vi "USRP oneTx_demoinfocom.vi"() -> ()   [LabVIEW 2021]
uses:
  system stop.vi
  <instrlib>/niUSRP/niUSRP Write Tx Data (CDB Cluster).vi
panel:
  out "Waveform Graph":dbl[](graph)
  in  "Duration":dbl format="%#_13g"
  in  "Frequency":dbl format="%#_13g"
  out "coerced carrier frequency":dbl=100000.0 format="%#_6p"
  out "coerced IQ rate":dbl=100000.0 format="%#_6p"
  in  "Tx IP":refnum<k15>
  in  "Tx Gain":dbl format="%#_6f"
  in  "carrier frequency":dbl=100000.0 format="%#_6p"
  in  "IQ rate":dbl=100000.0 format="%#_6p"
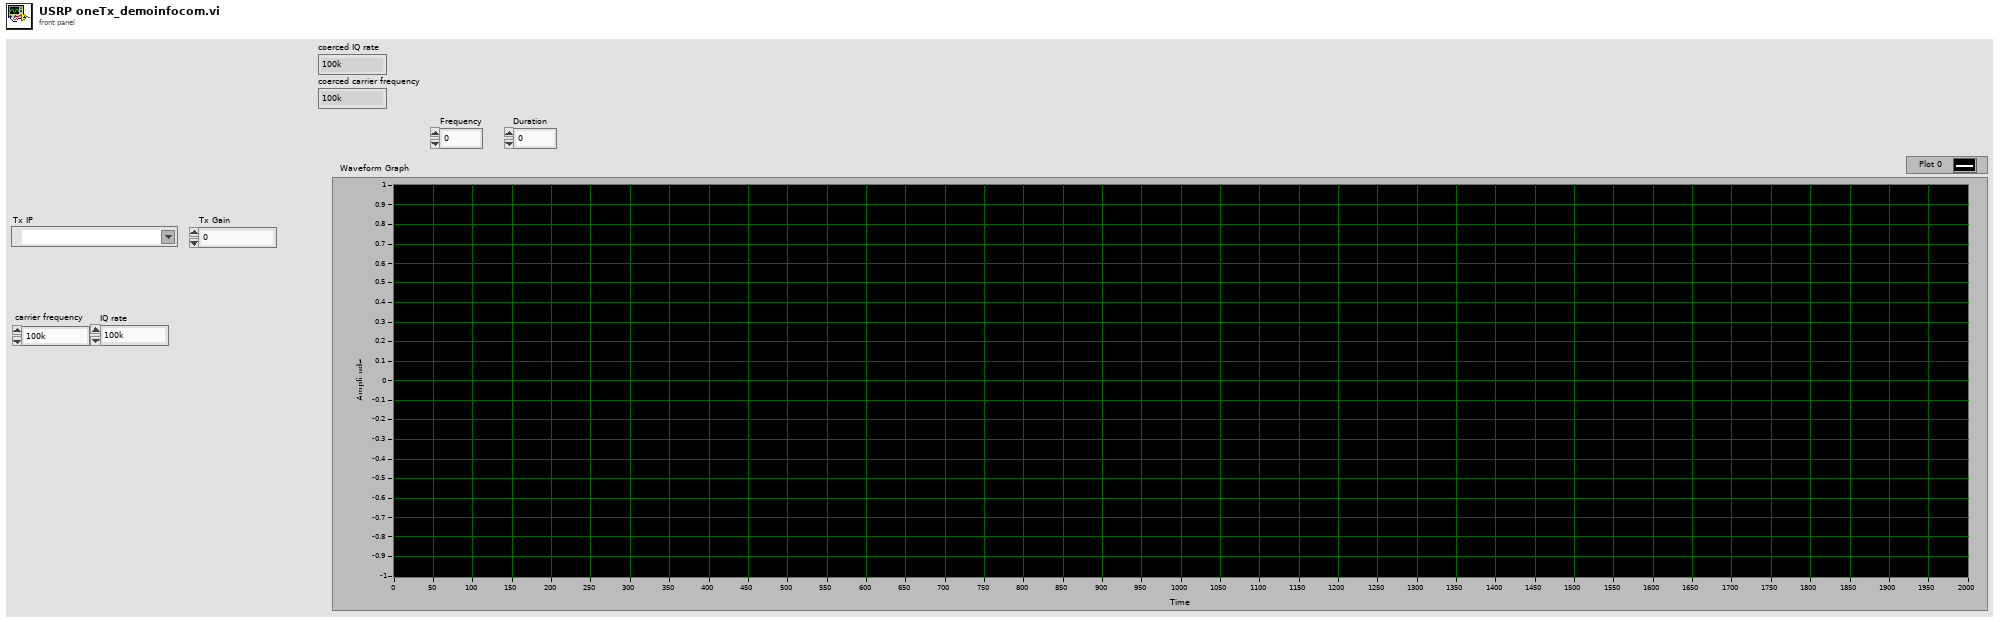
[diagram p1: front panel]
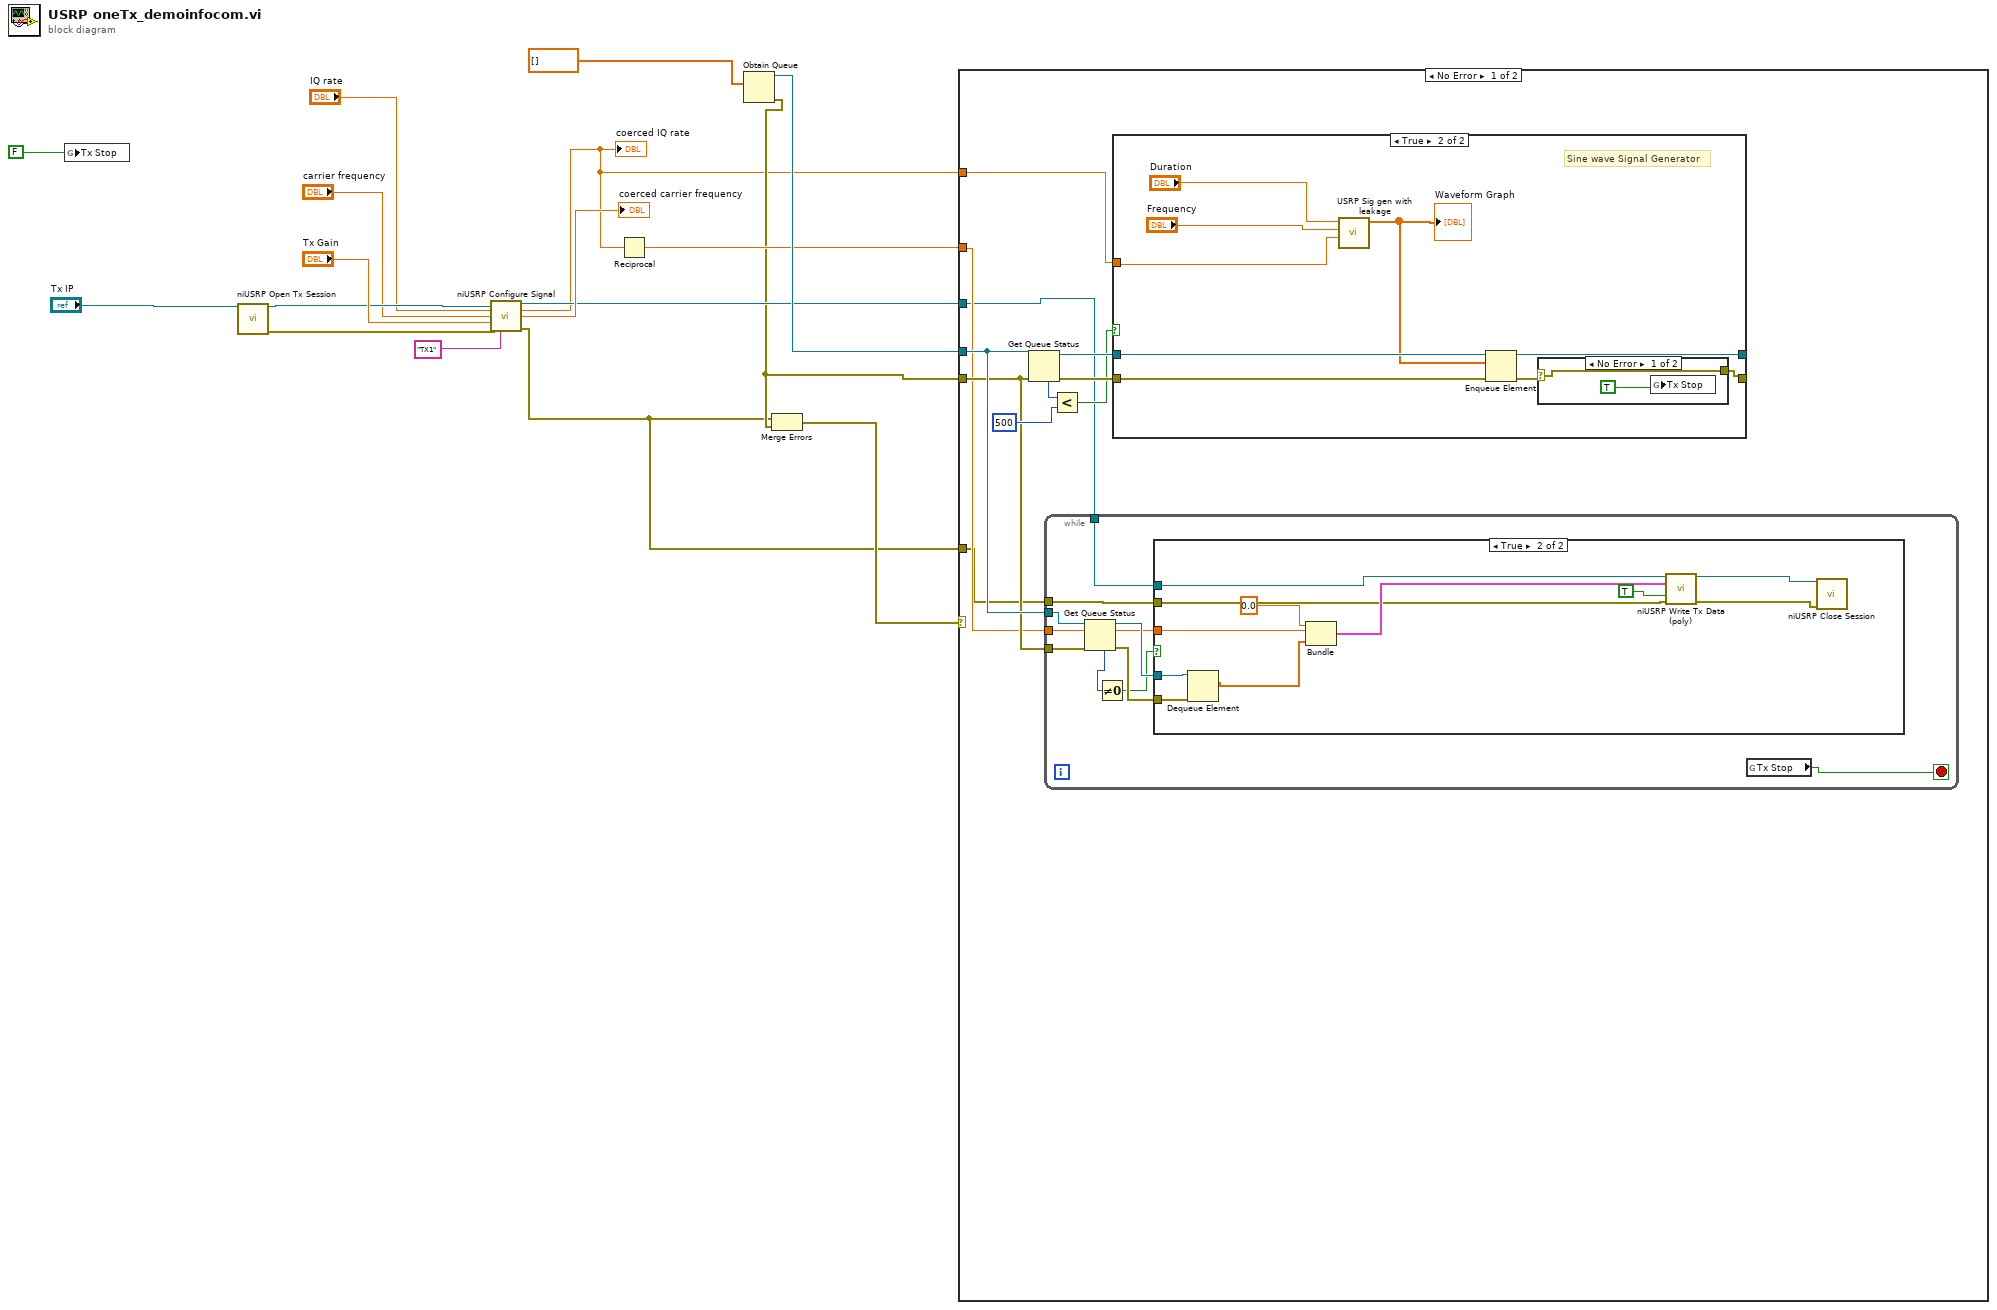
[diagram p0: block diagram]
diagram:
  n1 = global write "system stop.vi" "Tx Stop"(FALSE) -> ()
  n2 = call <instrlib>:"niUSRP Open Tx Session.vi"("device names"="Tx IP") -> ("session handle out"=w15:refnum<k15>, "error out"=w14:errorcluster)  [unwired: 13 in]
  n3 = call <instrlib>:"niUSRP Configure Signal.vi"("session handle"=w15, "IQ rate"="IQ rate", "carrier frequency"="carrier frequency", "gain"="Tx Gain", "error in (no error)"=w14, "active antenna"="TX1") -> ("session handle out"=w6:refnum<k15>, "coerced IQ rate"=w3:dbl, "coerced carrier frequency"=→"coerced carrier frequency":dbl, "error out"=w2:errorcluster)  [unwired: 5 in, 1 out]
  "coerced IQ rate" <- w3
  n4 = Reciprocal(x=w3) -> (1/x=w5:dbl)
  n5 = Obtain Queue(element data type=dbl[] []) -> (queue out=w7:refnum<queue>, error out=w4:errorcluster)  [unwired: 4 in, 1 out]
  n6 = Merge Errors(w2, w4) -> (w9:errorcluster)
  n7 = case shown="No Error" w9 {
    tunnel: w4 -> [w22 _]
    tunnel: w7 -> [w23 _]
    tunnel: w6 -> [w20 _]
    tunnel: w5 -> [w21 _]
    tunnel: w3 -> [w19 _]
    tunnel: w2 -> [w18 _]
    frame No Error {
      n8 = Get Queue Status(queue=w23, error in (no error)=w22) -> (queue out=w25:refnum<queue>, error out=w26:errorcluster, # elements in queue=w28:i32)  [unwired: 1 in, 5 out]
      n9 = while {
        tunnel: w23 -> [w38]
        tunnel: w22 -> [w35]
        tunnel: w21 -> [w34]
        tunnel: w20 -> [w32]
        tunnel: w18 -> [w29]
        stop <- w30 stop-if-true
        n10 = Get Queue Status(queue=w38, error in (no error)=w35) -> (queue out=w37:refnum<queue>, error out=w36:errorcluster, # elements in queue=w33:i32)  [unwired: 1 in, 5 out]
        n11 = Not Equal To 0?(x=w33) -> (x != 0?=w31:bool)
        n12 = case shown="True" w31 {
          tunnel: w37 -> [_ w49]
          tunnel: w36 -> [_ w48]
          tunnel: w34 -> [_ w47]
          tunnel: w32 -> [_ w45]
          tunnel: w29 -> [_ w40]
          frame False {
          }
          frame True {
            n13 = Dequeue Element(queue=w49, error in (no error)=w48) -> (element=w42:dbl[])  [unwired: 1 in, 3 out]
            n14 = Bundle(0.0, w47, w42) -> (w46:cluster{dbl, dbl, dbl[]})  [unwired: 1 in]
            n15 = call-poly <instrlib>:"niUSRP Write Tx Data (poly).vi"("session handle"=w45, "data"=w46, "end of data?"=TRUE, "error in (no error)"=w40) -> ("session handle out"=w44:refnum<k15>, "error out"=w43:errorcluster)  [unwired: 10 in]
            n16 = call <instrlib>:"niUSRP Close Session.vi"("session handle"=w44, "error in (no error)"=w43) -> ()  [unwired: 13 in, 1 out]
          }
        }
        n17 = global read "system stop.vi" "Tx Stop"() -> (w30:bool)
      }
      n18 = Less?(x=w28, y=500) -> (x < y?=w24:bool)
      n19 = case shown="True" w24 {
        tunnel: w26 -> [w50 w58]
        tunnel: w25 -> [w51 w57]
        tunnel: [w51 w56] -> _
        tunnel: [w50 w52] -> _
        tunnel: w19 -> [_ w54]
        frame False {
        }
        frame True {
          # "Sine wave Signal Generator"
          n20 = call "USRP Sig gen with leakage.vi"("Sampling rate"=w54, "Frequency"="Frequency", "Duration"="Duration") -> ("Array"=w55:dbl[])  [unwired: 7 in, 1 out]
          "Waveform Graph" <- w55
          n21 = Enqueue Element(queue=w57, element=w55, error in (no error)=w58) -> (queue out=w56:refnum<queue>, error out=w53:errorcluster)  [unwired: 1 in, 1 out]
          n22 = case shown="No Error" w53 {
            selector: w53 -> [w61 w63]
            tunnel: [w61 w63] -> w52
            frame No Error {
              n23 = global write "system stop.vi" "Tx Stop"(TRUE) -> ()
            }
            frame Error {
            }
          }
        }
      }
    }
    frame Error {
    }
  }
